vi "VeriStand DSF.Transfer Group.Configuration.Verify.Contiguous Engine Offsets.vi"(8 "error in (no error)":errorcluster, 11 "Transfer Group Configuration in":refnum<class "VeriStand DSF.Transfer Group.Configuration.lvclass">=refnum) -> (0 "error out":errorcluster, 3 "Transfer Group Configuration out":refnum<class "VeriStand DSF.Transfer Group.Configuration.lvclass">)   [LabVIEW 2017, in "Data Sharing Custom Device Engine.lvlib" / "VeriStand DSF.Transfer Group.Configuration.lvclass"]
uses:
  VeriStand DSF.Transfer Group.Configuration.lvclass
  Builds/Data Sharing Framework/Current/Data Sharing Framework Core/DSF Core.lvlibp/DSF Configuration API/Public/Controls/DSF Data Type.ctl
  Builds/Data Sharing Framework/Current/Data Sharing Framework Core/DSF Core.lvlibp/Shared/Classes/Transfer Group/Transfer Group Configuration.lvclass
  Builds/Data Sharing Framework/Current/Data Sharing Framework Core/DSF Core.lvlibp/Shared/Classes/Transfer/Transfer Configuration.lvclass
  Builds/Data Sharing Framework/Current/Data Sharing Framework Core/DSF Core.lvlibp
  C:/Builds/Data Sharing Framework/Current/Data Sharing Framework Core/DSF Core.lvlibp/Shared/Classes/Transfer Group/Transfer Group Configuration.lvclass
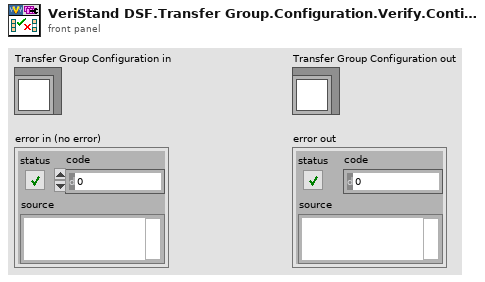
[diagram p1: front panel]
types:
  T1 = typedef "DSF Core.lvlibp/DSF Data Type.ctl" = enum8{"Bool", "SGL", "DBL", "I8", "I16", "I32", "I64", "U8", "U16", "U32", "U64"}
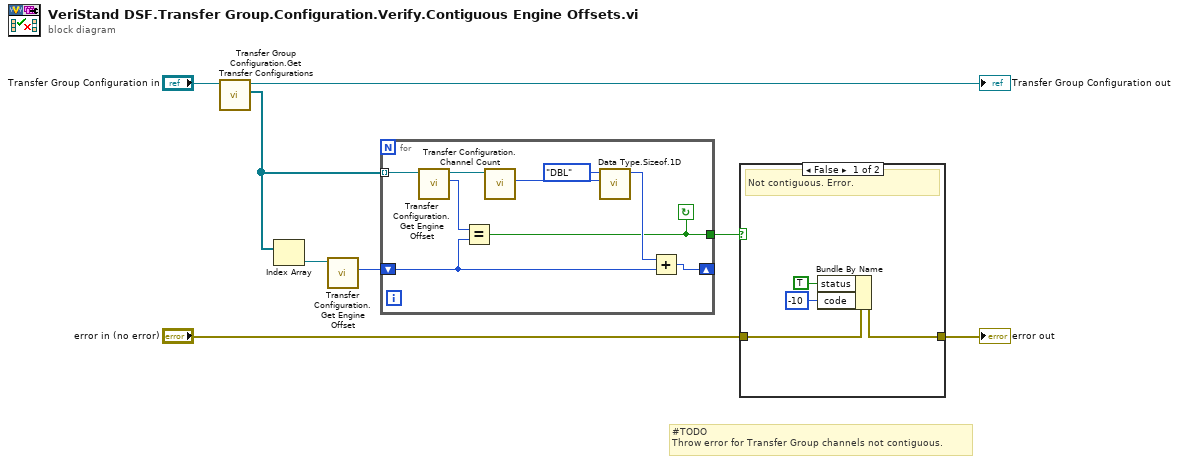
[diagram p0: block diagram]
diagram:
  # "#TODO\nThrow error for Transfer Group channels not contiguous."
  n1 = call "Transfer Group Configuration.Get Transfer Configurations.vi"("Transfer Group Configuration in"="Transfer Group Configuration in") -> ("Transfer Configurations"=w5:refnum<class "Transfer Configuration.lvclass">[], "Transfer Group Configuration out"=→"Transfer Group Configuration out":refnum<class "VeriStand DSF.Transfer Group.Configuration.lvclass">)  [unwired: 9 in]
  n2 = Index Array(array=w5) -> (element=w3:refnum<class "Transfer Configuration.lvclass">)  [unwired: 1 in]
  n3 = call "Transfer Configuration.Get Engine Offset.vi"("Transfer Configuration in"=w3) -> ("engine offset"=w4:u64)  [unwired: 9 in, 1 out]
  n4 = for {
    shift-right: [w11] -> _
    shift-left: w4 -> [w14]
    tunnel: w5 -> [w17] mode=indexing
    tunnel: [w10] -> w8
    stop <- w10 continue-if-true
    n5 = call "Transfer Configuration.Get Engine Offset.vi"("Transfer Configuration in"=w17) -> ("engine offset"=w15:u64, "Transfer Configuration out"=w16:refnum<class "Transfer Configuration.lvclass">)  [unwired: 9 in]
    n6 = Equal?(x=w15, y=w14) -> (x = y?=w10:bool)
    n7 = call "Transfer Configuration.Channel Count.vi"("Transfer Configuration in"=w16) -> ("total channel count"=w13:u64)  [unwired: 8 in, 2 out]
    n8 = call "Data Type.Sizeof.1D.vi"("count"=w13, "data type"=DSF_Data_Type."DBL") -> ("size in bytes"=w12:u64)  [unwired: 9 in]
    n9 = Add(x=w12, y=w14) -> (x+y=w11:u64)
  }
  n10 = case shown="False" w8 {
    tunnel: "error in (no error)" -> [w21 w22]
    tunnel: [w20 w22] -> w7
    frame False {
      # "Not contiguous. Error."
      n11 = Bundle By Name(cluster=w21, "status"=TRUE, "code"=-10) -> (w20:errorcluster)
    }
    frame True {
      # "Contiguous. Proceed."
    }
  }
  "error out" <- w7
